vi "Winch v5.vi"() -> ()   [LabVIEW 2013]
uses:
  Globals/Data for Dashboard.vi
  <vilib>/Rock Robotics/WPI/Joystick/WPI_JoystickGetSetRefNum.vi
  Robot Global Data.vi
  Globals/Useful Values.vi
  Globals/Homes.vi
  <vilib>/addons/control/pid/pid.llb/PID (DBL).vi
  <vilib>/Utility/file.llb/Write To Spreadsheet File (DBL).vi
  <vilib>/addons/control/pid/NI_PID_pid.lvlib
panel:
  out "Selector?":bool
  out "Winch Armed?":bool
  out "Winch Power":bool
  out "Full/half?":bool
  out "Full to Half?":bool
  out "Arm?":bool
  in  "PID gains":T1={"proportional gain (Kc)"=2.75, "integral time (Ti, min)"=0.0, "derivative time (Td, min)"=0.0} {"derivative time (Td, min)" format="%.3f"; "integral time (Ti, min)" format="%.3f"; "proportional gain (Kc)" format="%.3f"}
  # "PULLBACK SPEED NEEDS\nTO BE NEGATIVE OR ELSE"
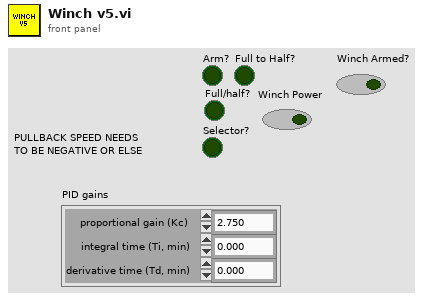
[diagram p1: front panel]
types:
  T1 = cluster{"proportional gain (Kc)":dbl, "integral time (Ti, min)":dbl, "derivative time (Td, min)":dbl}
  T2 = typedef "WPI_DigitalInputDevRef.ctl" = cluster{"DevStatus":errorcluster, "DIO Channel":T3, "Digital Module":T4}
  T3 = typedef "FPGA_DIOChannel.ctl" = enum8{"DIO 1", "DIO 2", "DIO 3", "DIO 4", "DIO 5", "DIO 6", "DIO 7", "DIO 8", "DIO 9", "DIO 10", "DIO 11", "DIO 12", "DIO 13", "DIO 14", "Invalid"}
  T4 = typedef "FPGA_TypedefDigitalModule.ctl" = enum16{"Digital Module 1", "Digital Module 2"}
  T5 = typedef "WPI_MotorControlDeviceRef.ctl" = cluster{"DeviceStatus":errorcluster, "Type":enum16{"PWM", "CAN"}, "PWM":cluster{"Digital Module":T4, "PWM Channel":T6, "DeadBand":T7}, "CAN":cluster{"Device Number":u8, "Control Mode":T8, "Semaphore":T9, "Max Vout":dbl}, "Invert":bool, "TransformRef":T10, "InvTransformRef":T10}
  T6 = typedef "FPGA_DIOPWMChannel.ctl" = enum8{"PWM 1", "PWM 2", "PWM 3", "PWM 4", "PWM 5", "PWM 6", "PWM 7", "PWM 8", "PWM 9", "PWM 10", "Invalid"}
  T7 = typedef "WPI_PWMDeadband.ctl" = cluster{"Name":string, "maxPositivePwm":i32, "minPositivePwm":i32, "centerPwm":i32, "maxNegativePwm":i32, "minNegativePwm":i32, "angularRange":u16}
  T8 = typedef "WPI_CANJaguar_ControlMode.ctl" = enum8{"Percent VBus", "Current", "Speed", "Position", "Voltage"}
  T9 = typedef "Semaphore RefNum" = refnum<k1>
  T10 = typedef "WPI_PWMTransform_ConPane.ctl" = refnum<vi>
  T11 = typedef "WPI_JoystickDevRef.ctl" = cluster{"Device":T12}
  T12 = typedef "WPI_JoystickDeviceEnum.ctl" = enum16{"USB 1", "USB 2", "USB 3", "USB 4", "Kinect 1", "Kinect 2"}
  T13 = typedef "WPI_AnalogChannelDevRef.ctl" = cluster{"DevStatus":errorcluster, "Analog Module":T14, "Analog Channel":T15}
  T14 = typedef "FPGA_TypedefAnalogModule.ctl" = enum16{"Analog Module 1", "Analog Module 2"}
  T15 = typedef "FPGA_AIChannel.ctl" = enum8{"AI 1", "AI 2", "AI 3", "AI 4", "AI 5", "AI 6", "AI 7", "AI 8", "Invalid"}
  T16 = typedef "WPI_DriverStationRobotMode2.ctl" = enum16{"Autonomous Disabled", "Autonomous Enabled", "Teleop Disabled", "Teleop Enabled", "Timeout", "Finish", "Test Disabled", "Test Enabled"}
  T17 = typedef "WPI_JoystickButtonState.ctl" = cluster{"Button 1":bool, "Button 2":bool, "Button 3":bool, "Button 4":bool, "Button 5":bool, "Button 6":bool, "Button 7":bool, "Button 8":bool, "Button 9":bool, "Button 10":bool, "Button 11":bool, "Button 12":bool}
  T18 = cluster{"axis 1 (x)":dbl, "axis 2 (y)":dbl, "axis 3 (throttle)":dbl, "axis 4":dbl, "axis 5":dbl, "axis 6":dbl}
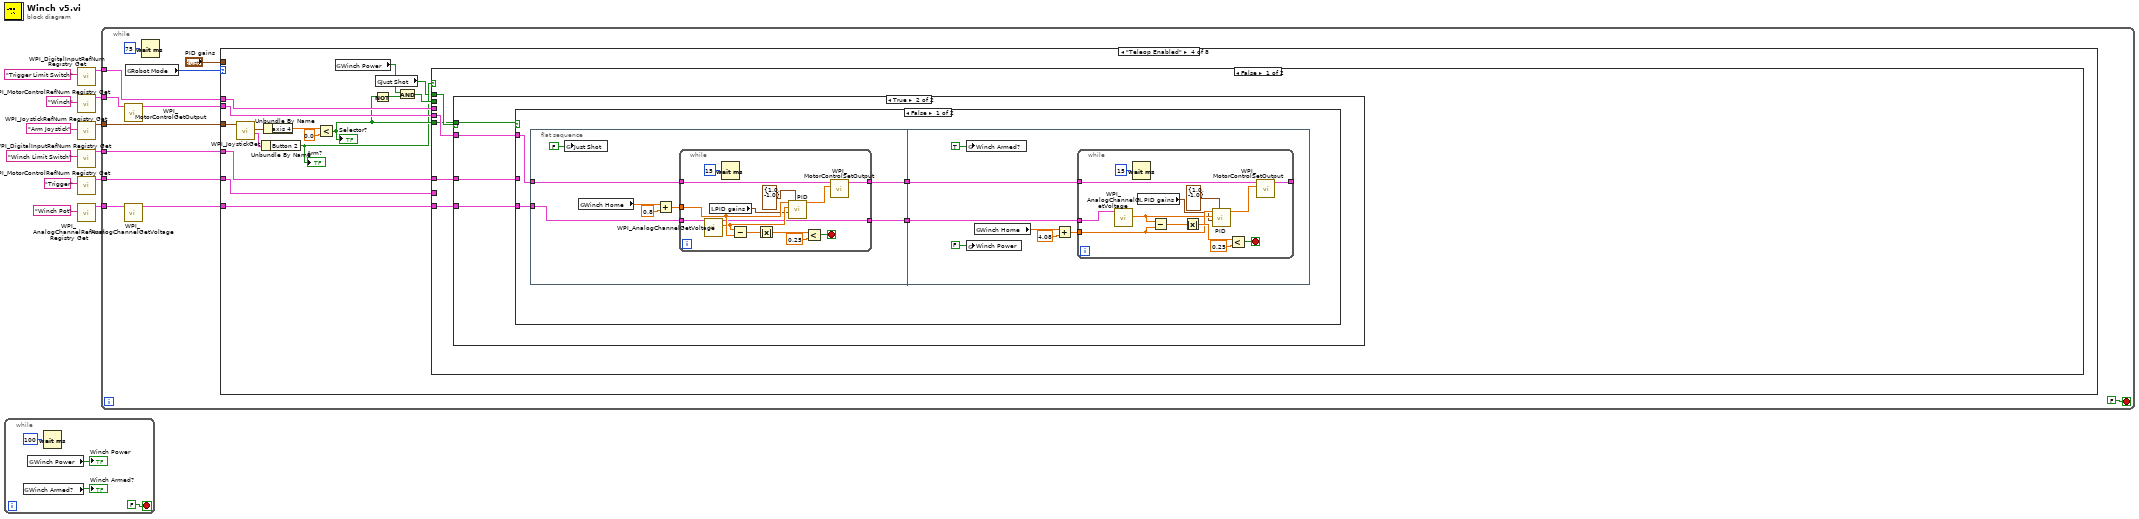
[diagram p0: block diagram]
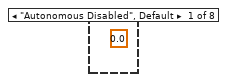
[diagram p2: hidden frame]
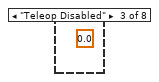
[diagram p4: hidden frame]
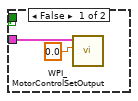
[diagram p5: hidden frame]
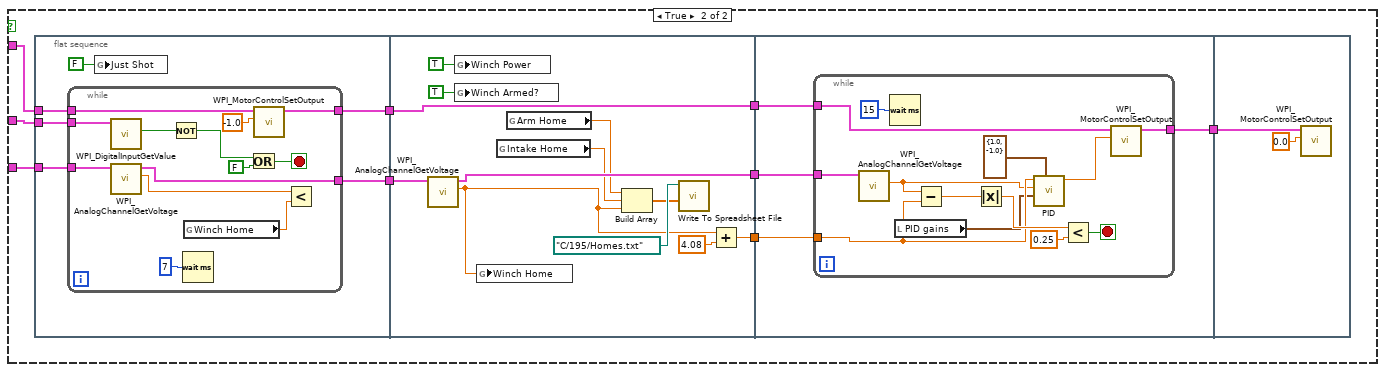
[diagram p6: hidden frame]
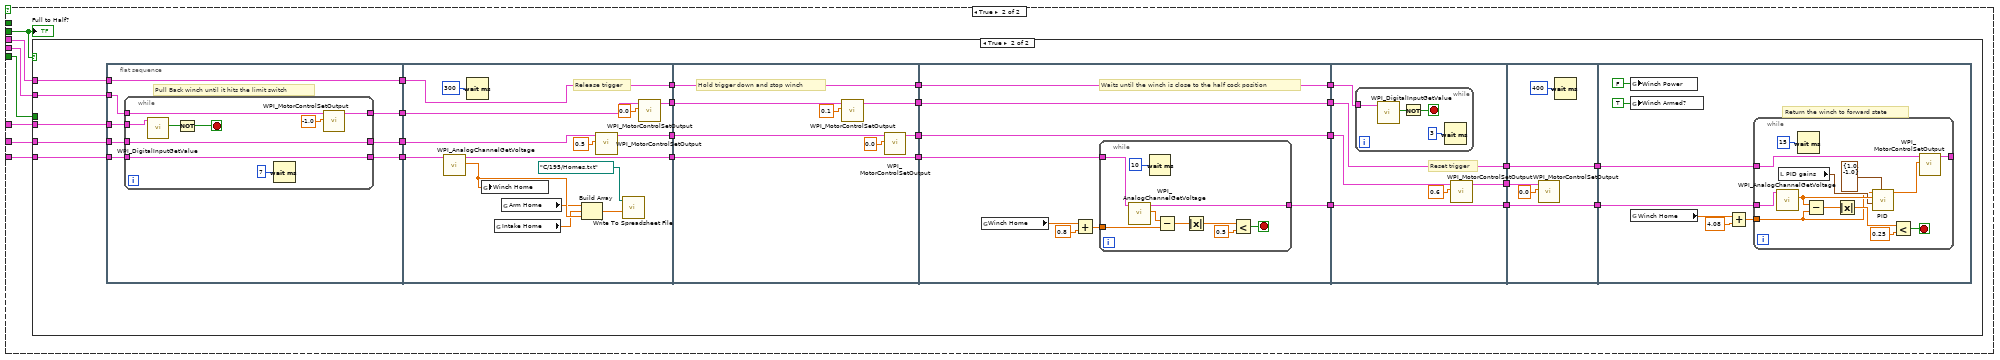
[diagram p7: hidden frame]
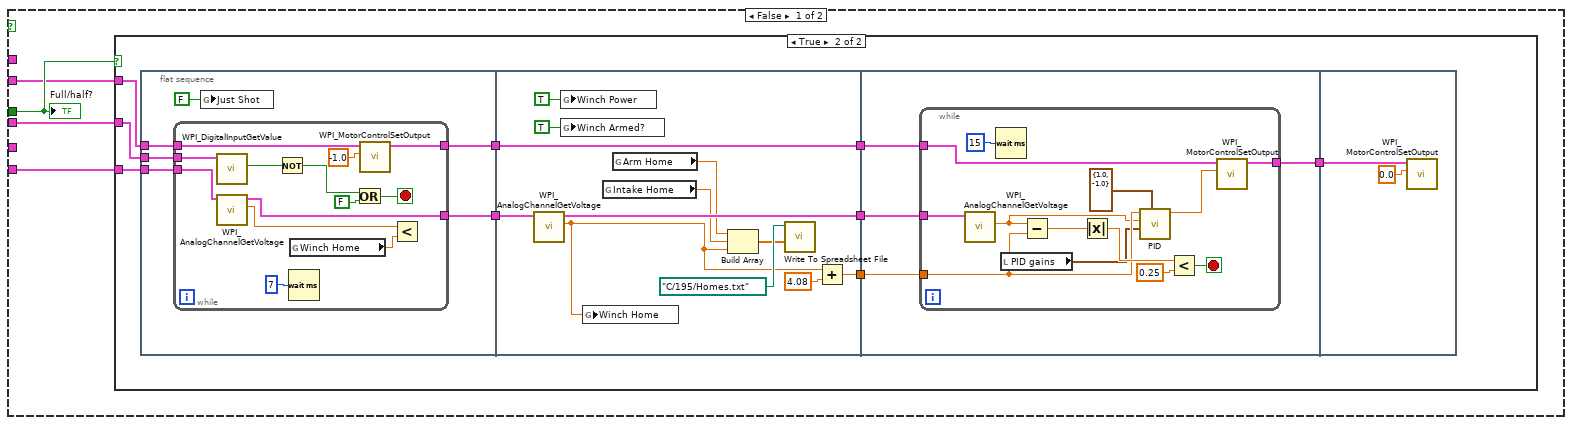
[diagram p8: hidden frame]
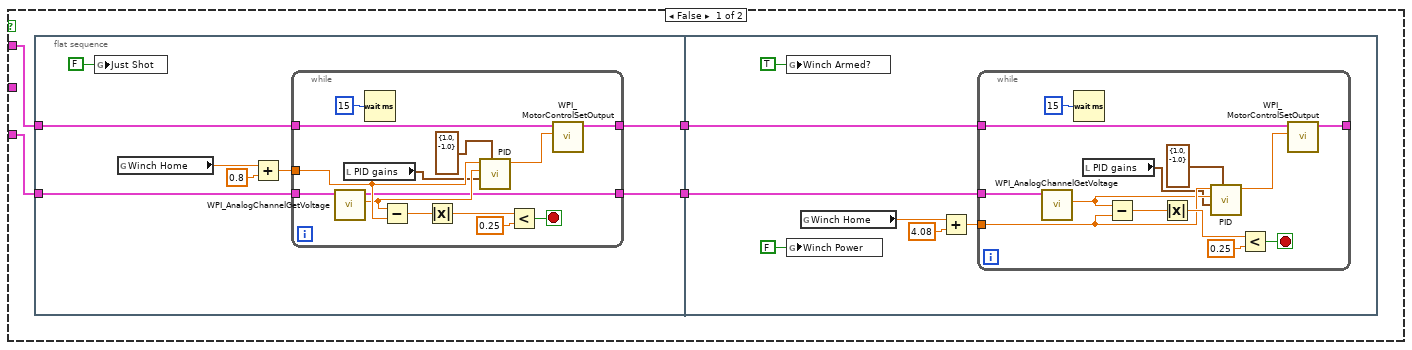
[diagram p9: hidden frame]
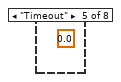
[diagram p10: hidden frame]
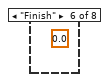
[diagram p11: hidden frame]
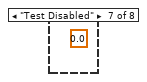
[diagram p12: hidden frame]
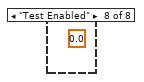
[diagram p13: hidden frame]
diagram:
  n1 = while {
    stop <- FALSE stop-if-true
    n2 = global read "Data for Dashboard.vi" "Winch Armed?"() -> (→"Winch Armed?":bool)
    n3 = global read "Data for Dashboard.vi" "Winch Power"() -> (→"Winch Power":bool)
    n4 = Wait (ms)(milliseconds to wait=u32 100) -> ()  [unwired: 1 out]
  }
  n5 = call <vilib>:"WPI_DigitalInputRefNum Registry Get.vi"("refnum name"="Trigger Limit Switch") -> ("DigitalInputDevRef"=w1:T2)  [unwired: 9 in, 1 out]
  n6 = call <vilib>:"WPI_MotorControlRefNum Registry Get.vi"("refnum name"="Winch") -> ("MotorControlDevRef"=w9:T5)  [unwired: 9 in, 1 out]
  n7 = call <vilib>:"WPI_JoystickRefNum Registry Get.vi"("refnum name"="Arm Joystick") -> ("JoystickDevRef"=w7:T11)  [unwired: 9 in, 1 out]
  n8 = call <vilib>:"WPI_DigitalInputRefNum Registry Get.vi"("refnum name"="Winch Limit Switch") -> ("DigitalInputDevRef"=w6:T2)  [unwired: 9 in, 1 out]
  n9 = call <vilib>:"WPI_MotorControlRefNum Registry Get.vi"("refnum name"="Trigger") -> ("MotorControlDevRef"=w3:T5)  [unwired: 9 in, 1 out]
  n10 = call <vilib>:"WPI_AnalogChannelRefNum Registry Get.vi"("refnum name"="Winch Pot") -> ("AIDeviceRef"=w12:T13)  [unwired: 9 in, 1 out]
  n11 = while {
    tunnel: w12 -> [w26]
    tunnel: w9 -> [w21]
    tunnel: w7 -> [w23]
    tunnel: w6 -> [w18]
    tunnel: w3 -> [w19]
    tunnel: w1 -> [w17]
    stop <- FALSE stop-if-true
    n12 = call <vilib>:"WPI_MotorControlGetOutput.vi"("MotorControlDevRef"=w21) -> ("MotorControlDevRef"=w20:T5)  [unwired: 8 in, 2 out]
    n13 = call <vilib>:"WPI_AnalogChannelGetVoltage.vi"("AIDeviceRef"=w26) -> ("AIDeviceRef"=w22:T13)  [unwired: 8 in, 2 out]
    n14 = global read "Robot Global Data.vi" "Robot Mode"() -> (w25:T16)
    n15 = Wait (ms)(milliseconds to wait=u32 75) -> ()  [unwired: 1 out]
    n16 = case shown="\"Teleop Enabled\"" w25 {
      tunnel: w20 -> [_ _ _ w41 _ _ _ _]
      tunnel: "PID gains" -> [_ _ _ _ _ _ _ _]
      tunnel: w23 -> [_ _ _ w44 _ _ _ _]
      tunnel: w18 -> [_ _ _ w42 _ _ _ _]
      tunnel: w22 -> [_ _ _ w40 _ _ _ _]
      tunnel: w19 -> [_ _ _ w39 _ _ _ _]
      tunnel: w17 -> [_ _ _ w38 _ _ _ _]
      frame "Autonomous Disabled", Default {
        (unwired) 0.0 ("Motor Output")
      }
      frame "Autonomous Enabled" {
      }
      frame "Teleop Disabled" {
        (unwired) 0.0 ("Motor Output")
      }
      frame "Teleop Enabled" {
        n17 = call <vilib>:"WPI_JoystickGet.vi"("JoystickDevRef"=w44) -> ("Buttons"=w43:T17, "Axes"=w35:T18)  [unwired: 4 in, 1 out]
        n18 = Unbundle By Name(w43) -> ("Button 2"=w30:bool)
        "Arm?" <- w30
        n19 = Unbundle By Name(w35) -> ("axis 4"=w34:dbl)
        n20 = Less?(x=w34, y=0.0) -> (x < y?=w32:bool)
        "Selector?" <- w32
        n21 = global read "Data for Dashboard.vi" "Winch Power"() -> (w36:bool)
        n22 = Not(x=w32) -> (.not. x?=w31:bool)
        n23 = global read "Useful Values.vi" "Just Shot"() -> (w29:bool)
        n24 = And(x=w36, y=w31) -> (x .and. y?=w37:bool)
        n25 = case shown="False" w30 {
          tunnel: w42 -> [w47 w165]
          tunnel: w41 -> [w49 w167]
          tunnel: w40 -> [w46 w166]
          tunnel: w39 -> [_ w164]
          tunnel: w38 -> [_ w163]
          tunnel: w37 -> [_ w162]
          tunnel: w32 -> [w45 w161]
          tunnel: w29 -> [w48 _]
          frame False {
            n26 = case shown="True" w48 {
              tunnel: w49 -> [w51 w54]
              tunnel: w47 -> [_ w55]
              tunnel: w46 -> [_ w53]
              tunnel: w45 -> [_ w52]
              frame False {
                n27 = call <vilib>:"WPI_MotorControlSetOutput.vi"("Output"=0.0, "MotorControlDevRef"=w51) -> ()  [unwired: 7 in, 3 out]
              }
              frame True {
                n28 = case shown="False" w52 {
                  tunnel: w54 -> [w58 w104]
                  tunnel: w53 -> [w59 w103]
                  tunnel: w55 -> [_ w102]
                  frame False {
                    n29 = flat-sequence {
                      tunnel: w58 -> [w67]
                      tunnel: w59 -> [w66]
                      tunnel: [w62] -> w57
                      tunnel: [w61] -> w56
                      tunnel: w57 -> [w88]
                      tunnel: w56 -> [w87]
                      frame #0 {
                        n30 = global write "Useful Values.vi" "Just Shot"(FALSE ("Just Shot")) -> ()
                        n31 = global read "Homes.vi" "Winch Home"() -> (w65:dbl)
                        n32 = Add(x=w65, y=0.8) -> (x+y=w63:dbl)
                        n33 = while {
                          tunnel: w67 -> [w81]
                          tunnel: w63 -> [w74]
                          tunnel: w66 -> [w76]
                          tunnel: [w72] -> w62
                          tunnel: [w68] -> w61
                          stop <- w78 stop-if-true
                          n34 = call <vilib>:"WPI_AnalogChannelGetVoltage.vi"("AIDeviceRef"=w76) -> ("Voltage"=w73:dbl, "AIDeviceRef"=w68:T13)  [unwired: 8 in, 1 out]
                          n35 = local read "PID gains"() -> (w71:T1)
                          n36 = Wait (ms)(milliseconds to wait=u32 15) -> ()  [unwired: 1 out]
                          n37 = Subtract(x=w73, y=w74) -> (x-y=w80:dbl)
                          n38 = Absolute Value(x=w80) -> (abs(x)=w79:dbl)
                          n39 = call-poly <vilib>:"PID.vi"("output range"=cluster{"output high":dbl, "output low":dbl} {"output high"=1.0, "output low"=-1.0}, "PID gains"=w71, "process variable"=w73, "setpoint"=w74) -> ("output"=w69:dbl)  [unwired: 6 in, 1 out]
                          n40 = Less?(x=w79, y=0.25) -> (x < y?=w78:bool)
                          n41 = call <vilib>:"WPI_MotorControlSetOutput.vi"("Output"=w69, "MotorControlDevRef"=w81) -> ("MotorControlDevRef"=w72:T5)  [unwired: 7 in, 2 out]
                        }
                      }
                      frame #1 {
                        n42 = global write "Data for Dashboard.vi" "Winch Armed?"(TRUE ("Loaded")) -> ()
                        n43 = global write "Data for Dashboard.vi" "Winch Power"(FALSE ("Loaded")) -> ()
                        n44 = global read "Homes.vi" "Winch Home"() -> (w86:dbl)
                        n45 = Add(x=w86, y=4.08) -> (x+y=w84:dbl)
                        n46 = while {
                          tunnel: w88 -> [w101]
                          tunnel: w84 -> [w94]
                          tunnel: w87 -> [w96]
                          tunnel: [w92] -> _
                          stop <- w98 stop-if-true
                          n47 = call <vilib>:"WPI_AnalogChannelGetVoltage.vi"("AIDeviceRef"=w96) -> ("Voltage"=w93:dbl)  [unwired: 8 in, 2 out]
                          n48 = Wait (ms)(milliseconds to wait=u32 15) -> ()  [unwired: 1 out]
                          n49 = local read "PID gains"() -> (w91:T1)
                          n50 = Subtract(x=w93, y=w94) -> (x-y=w100:dbl)
                          n51 = Absolute Value(x=w100) -> (abs(x)=w99:dbl)
                          n52 = call-poly <vilib>:"PID.vi"("output range"=cluster{"output high":dbl, "output low":dbl} {"output high"=1.0, "output low"=-1.0}, "PID gains"=w91, "process variable"=w93, "setpoint"=w94) -> ("output"=w89:dbl)  [unwired: 6 in, 1 out]
                          n53 = Less?(x=w99, y=0.25) -> (x < y?=w98:bool)
                          n54 = call <vilib>:"WPI_MotorControlSetOutput.vi"("Output"=w89, "MotorControlDevRef"=w101) -> ("MotorControlDevRef"=w92:T5)  [unwired: 7 in, 2 out]
                        }
                      }
                    }
                  }
                  frame True {
                    n55 = flat-sequence {
                      tunnel: w102 -> [w116]
                      tunnel: w104 -> [w115]
                      tunnel: [w114] -> w110
                      tunnel: [w111] -> w109
                      tunnel: w103 -> [w112]
                      tunnel: w110 -> [w141]
                      tunnel: [w141] -> w108
                      tunnel: [w140] -> w107
                      tunnel: w109 -> [w139]
                      tunnel: [w138] -> w106
                      tunnel: w108 -> [w145]
                      tunnel: w107 -> [w143]
                      tunnel: [w142] -> w105
                      tunnel: w106 -> [w144]
                      tunnel: w105 -> [w160]
                      frame #0 {
                        n56 = while {
                          tunnel: w116 -> [w129]
                          tunnel: w115 -> [w125]
                          tunnel: [w124] -> w114
                          tunnel: w112 -> [w123]
                          tunnel: [w122] -> w111
                          stop <- w119 stop-if-true
                          n57 = call <vilib>:"WPI_DigitalInputGetValue.vi"("DigitalInputDevRef"=w129) -> ("Value"=w128:bool)  [unwired: 8 in, 2 out]
                          n58 = call <vilib>:"WPI_AnalogChannelGetVoltage.vi"("AIDeviceRef"=w123) -> ("Voltage"=w121:dbl, "AIDeviceRef"=w122:T13)  [unwired: 8 in, 1 out]
                          n59 = Not(x=w128) -> (.not. x?=w118:bool)
                          n60 = Wait (ms)(milliseconds to wait=u32 7) -> ()  [unwired: 1 out]
                          n61 = global read "Homes.vi" "Winch Home"() -> (w120:dbl)
                          n62 = Or(x=w118, y=FALSE) -> (x .or. y?=w119:bool)
                          n63 = call <vilib>:"WPI_MotorControlSetOutput.vi"("Output"=-1.0 ("Pullback Speed"), "MotorControlDevRef"=w125) -> ("MotorControlDevRef"=w124:T5)  [unwired: 7 in, 2 out]
                          n64 = Less?(x=w121, y=w120) -> ()  [unwired: 1 out]
                        }
                        n65 = global write "Useful Values.vi" "Just Shot"(FALSE ("Just Shot")) -> ()
                      }
                      frame #1 {
                        n66 = call <vilib>:"WPI_AnalogChannelGetVoltage.vi"("AIDeviceRef"=w139) -> ("Voltage"=w132:dbl, "AIDeviceRef"=w140:T13)  [unwired: 8 in, 1 out]
                        n67 = global write "Data for Dashboard.vi" "Winch Power"(TRUE ("Loaded")) -> ()
                        n68 = global write "Data for Dashboard.vi" "Winch Armed?"(TRUE ("Loaded")) -> ()
                        n69 = global write "Homes.vi" "Winch Home"(w132) -> ()
                        n70 = global read "Homes.vi" "Intake Home"() -> (w133:dbl)
                        n71 = global read "Homes.vi" "Arm Home"() -> (w135:dbl)
                        n72 = Build Array(w135, w133, w132) -> (w134:dbl[])
                        n73 = call-poly <vilib>:"Write To Spreadsheet File.vi"("1D data"=w134, "file path (dialog if empty)"=path "C:/195/Homes.txt") -> ()  [unwired: 6 in, 1 out]
                        n74 = Add(x=w132, y=4.08) -> (x+y=w138:dbl)
                      }
                      frame #2 {
                        n75 = while {
                          tunnel: w145 -> [w158]
                          tunnel: w144 -> [w151]
                          tunnel: w143 -> [w153]
                          tunnel: [w149] -> w142
                          stop <- w155 stop-if-true
                          n76 = call <vilib>:"WPI_AnalogChannelGetVoltage.vi"("AIDeviceRef"=w153) -> ("Voltage"=w150:dbl)  [unwired: 8 in, 2 out]
                          n77 = Wait (ms)(milliseconds to wait=u32 15) -> ()  [unwired: 1 out]
                          n78 = local read "PID gains"() -> (w148:T1)
                          n79 = Subtract(x=w150, y=w151) -> (x-y=w157:dbl)
                          n80 = Absolute Value(x=w157) -> (abs(x)=w156:dbl)
                          n81 = call-poly <vilib>:"PID.vi"("output range"=cluster{"output high":dbl, "output low":dbl} {"output high"=1.0, "output low"=-1.0}, "PID gains"=w148, "process variable"=w150, "setpoint"=w151) -> ("output"=w146:dbl)  [unwired: 6 in, 1 out]
                          n82 = Less?(x=w156, y=0.25) -> (x < y?=w155:bool)
                          n83 = call <vilib>:"WPI_MotorControlSetOutput.vi"("Output"=w146, "MotorControlDevRef"=w158) -> ("MotorControlDevRef"=w149:T5)  [unwired: 7 in, 2 out]
                        }
                      }
                      frame #3 {
                        n84 = call <vilib>:"WPI_MotorControlSetOutput.vi"("Output"=0.0, "MotorControlDevRef"=w160) -> ()  [unwired: 7 in, 3 out]
                      }
                    }
                  }
                }
              }
            }
          }
          frame True {
            n85 = case shown="True" w162 {
              tunnel: w167 -> [w170 w281]
              tunnel: w166 -> [w169 w280]
              tunnel: w165 -> [w168 w279]
              tunnel: w164 -> [_ w278]
              tunnel: w163 -> [_ w277]
              tunnel: w161 -> [w171 _]
              frame False {
                n86 = case shown="True" w171 {
                  tunnel: w170 -> [w174 w220]
                  tunnel: w169 -> [w175 w219]
                  tunnel: w168 -> [_ w218]
                  frame False {
                    n87 = flat-sequence {
                      tunnel: w174 -> [w183]
                      tunnel: w175 -> [w182]
                      tunnel: [w178] -> w173
                      tunnel: [w177] -> w172
                      tunnel: w173 -> [w204]
                      tunnel: w172 -> [w203]
                      frame #0 {
                        n88 = global write "Useful Values.vi" "Just Shot"(FALSE ("Just Shot")) -> ()
                        n89 = global read "Homes.vi" "Winch Home"() -> (w181:dbl)
                        n90 = Add(x=w181, y=0.8) -> (x+y=w179:dbl)
                        n91 = while {
                          tunnel: w183 -> [w197]
                          tunnel: w179 -> [w190]
                          tunnel: w182 -> [w192]
                          tunnel: [w188] -> w178
                          tunnel: [w184] -> w177
                          stop <- w194 stop-if-true
                          n92 = call <vilib>:"WPI_AnalogChannelGetVoltage.vi"("AIDeviceRef"=w192) -> ("Voltage"=w189:dbl, "AIDeviceRef"=w184:T13)  [unwired: 8 in, 1 out]
                          n93 = local read "PID gains"() -> (w187:T1)
                          n94 = Wait (ms)(milliseconds to wait=u32 15) -> ()  [unwired: 1 out]
                          n95 = Subtract(x=w189, y=w190) -> (x-y=w196:dbl)
                          n96 = Absolute Value(x=w196) -> (abs(x)=w195:dbl)
                          n97 = call-poly <vilib>:"PID.vi"("output range"=cluster{"output high":dbl, "output low":dbl} {"output high"=1.0, "output low"=-1.0}, "PID gains"=w187, "process variable"=w189, "setpoint"=w190) -> ("output"=w185:dbl)  [unwired: 6 in, 1 out]
                          n98 = Less?(x=w195, y=0.25) -> (x < y?=w194:bool)
                          n99 = call <vilib>:"WPI_MotorControlSetOutput.vi"("Output"=w185, "MotorControlDevRef"=w197) -> ("MotorControlDevRef"=w188:T5)  [unwired: 7 in, 2 out]
                        }
                      }
                      frame #1 {
                        n100 = global write "Data for Dashboard.vi" "Winch Armed?"(TRUE ("Loaded")) -> ()
                        n101 = global write "Data for Dashboard.vi" "Winch Power"(FALSE ("Loaded")) -> ()
                        n102 = global read "Homes.vi" "Winch Home"() -> (w202:dbl)
                        n103 = Add(x=w202, y=4.08) -> (x+y=w200:dbl)
                        n104 = while {
                          tunnel: w204 -> [w217]
                          tunnel: w200 -> [w210]
                          tunnel: w203 -> [w212]
                          tunnel: [w208] -> _
                          stop <- w214 stop-if-true
                          n105 = call <vilib>:"WPI_AnalogChannelGetVoltage.vi"("AIDeviceRef"=w212) -> ("Voltage"=w209:dbl)  [unwired: 8 in, 2 out]
                          n106 = Wait (ms)(milliseconds to wait=u32 15) -> ()  [unwired: 1 out]
                          n107 = local read "PID gains"() -> (w207:T1)
                          n108 = Subtract(x=w209, y=w210) -> (x-y=w216:dbl)
                          n109 = Absolute Value(x=w216) -> (abs(x)=w215:dbl)
                          n110 = call-poly <vilib>:"PID.vi"("output range"=cluster{"output high":dbl, "output low":dbl} {"output high"=1.0, "output low"=-1.0}, "PID gains"=w207, "process variable"=w209, "setpoint"=w210) -> ("output"=w205:dbl)  [unwired: 6 in, 1 out]
                          n111 = Less?(x=w215, y=0.25) -> (x < y?=w214:bool)
                          n112 = call <vilib>:"WPI_MotorControlSetOutput.vi"("Output"=w205, "MotorControlDevRef"=w217) -> ("MotorControlDevRef"=w208:T5)  [unwired: 7 in, 2 out]
                        }
                      }
                    }
                  }
                  frame True {
                    n113 = flat-sequence {
                      tunnel: w218 -> [w232]
                      tunnel: w220 -> [w231]
                      tunnel: [w230] -> w226
                      tunnel: [w227] -> w225
                      tunnel: w219 -> [w228]
                      tunnel: w226 -> [w257]
                      tunnel: [w257] -> w224
                      tunnel: [w256] -> w223
                      tunnel: w225 -> [w255]
                      tunnel: [w254] -> w222
                      tunnel: w224 -> [w261]
                      tunnel: w223 -> [w259]
                      tunnel: [w258] -> w221
                      tunnel: w222 -> [w260]
                      tunnel: w221 -> [w276]
                      frame #0 {
                        n114 = while {
                          tunnel: w232 -> [w245]
                          tunnel: w231 -> [w241]
                          tunnel: [w240] -> w230
                          tunnel: w228 -> [w239]
                          tunnel: [w238] -> w227
                          stop <- w235 stop-if-true
                          n115 = call <vilib>:"WPI_DigitalInputGetValue.vi"("DigitalInputDevRef"=w245) -> ("Value"=w244:bool)  [unwired: 8 in, 2 out]
                          n116 = call <vilib>:"WPI_AnalogChannelGetVoltage.vi"("AIDeviceRef"=w239) -> ("Voltage"=w237:dbl, "AIDeviceRef"=w238:T13)  [unwired: 8 in, 1 out]
                          n117 = Not(x=w244) -> (.not. x?=w234:bool)
                          n118 = Wait (ms)(milliseconds to wait=u32 7) -> ()  [unwired: 1 out]
                          n119 = global read "Homes.vi" "Winch Home"() -> (w236:dbl)
                          n120 = Or(x=w234, y=FALSE) -> (x .or. y?=w235:bool)
                          n121 = call <vilib>:"WPI_MotorControlSetOutput.vi"("Output"=-1.0 ("Pullback Speed"), "MotorControlDevRef"=w241) -> ("MotorControlDevRef"=w240:T5)  [unwired: 7 in, 2 out]
                          n122 = Less?(x=w237, y=w236) -> ()  [unwired: 1 out]
                        }
                        n123 = global write "Useful Values.vi" "Just Shot"(FALSE ("Just Shot")) -> ()
                      }
                      frame #1 {
                        n124 = call <vilib>:"WPI_AnalogChannelGetVoltage.vi"("AIDeviceRef"=w255) -> ("Voltage"=w248:dbl, "AIDeviceRef"=w256:T13)  [unwired: 8 in, 1 out]
                        n125 = global write "Data for Dashboard.vi" "Winch Power"(TRUE ("Loaded")) -> ()
                        n126 = global write "Data for Dashboard.vi" "Winch Armed?"(TRUE ("Loaded")) -> ()
                        n127 = global write "Homes.vi" "Winch Home"(w248) -> ()
                        n128 = global read "Homes.vi" "Intake Home"() -> (w249:dbl)
                        n129 = global read "Homes.vi" "Arm Home"() -> (w251:dbl)
                        n130 = Build Array(w251, w249, w248) -> (w250:dbl[])
                        n131 = call-poly <vilib>:"Write To Spreadsheet File.vi"("1D data"=w250, "file path (dialog if empty)"=path "C:/195/Homes.txt") -> ()  [unwired: 6 in, 1 out]
                        n132 = Add(x=w248, y=4.08) -> (x+y=w254:dbl)
                      }
                      frame #2 {
                        n133 = while {
                          tunnel: w261 -> [w274]
                          tunnel: w260 -> [w267]
                          tunnel: w259 -> [w269]
                          tunnel: [w265] -> w258
                          stop <- w271 stop-if-true
                          n134 = call <vilib>:"WPI_AnalogChannelGetVoltage.vi"("AIDeviceRef"=w269) -> ("Voltage"=w266:dbl)  [unwired: 8 in, 2 out]
                          n135 = Wait (ms)(milliseconds to wait=u32 15) -> ()  [unwired: 1 out]
                          n136 = local read "PID gains"() -> (w264:T1)
                          n137 = Subtract(x=w266, y=w267) -> (x-y=w273:dbl)
                          n138 = Absolute Value(x=w273) -> (abs(x)=w272:dbl)
                          n139 = call-poly <vilib>:"PID.vi"("output range"=cluster{"output high":dbl, "output low":dbl} {"output high"=1.0, "output low"=-1.0}, "PID gains"=w264, "process variable"=w266, "setpoint"=w267) -> ("output"=w262:dbl)  [unwired: 6 in, 1 out]
                          n140 = Less?(x=w272, y=0.25) -> (x < y?=w271:bool)
                          n141 = call <vilib>:"WPI_MotorControlSetOutput.vi"("Output"=w262, "MotorControlDevRef"=w274) -> ("MotorControlDevRef"=w265:T5)  [unwired: 7 in, 2 out]
                        }
                      }
                      frame #3 {
                        n142 = call <vilib>:"WPI_MotorControlSetOutput.vi"("Output"=0.0, "MotorControlDevRef"=w276) -> ()  [unwired: 7 in, 3 out]
                      }
                    }
                  }
                }
                "Full/half?" <- w171
              }
              frame True {
                n143 = flat-sequence {
                  tunnel: w281 -> [w310]
                  tunnel: w280 -> [w309]
                  tunnel: w279 -> [w308]
                  tunnel: w278 -> [w306]
                  tunnel: [w307] -> w302
                  tunnel: [w305] -> w301
                  tunnel: [w304] -> w300
                  tunnel: [w303] -> w299
                  tunnel: w277 -> [w303]
                  tunnel: w302 -> [w334]
                  tunnel: [w331] -> w298
                  tunnel: [w320] -> w297
                  tunnel: w301 -> [w322]
                  tunnel: w300 -> [w324]
                  tunnel: [w323] -> w296
                  tunnel: [w330] -> w295
                  tunnel: w299 -> [w330]
                  tunnel: w298 -> [w342]
                  tunnel: w297 -> [w339]
                  tunnel: w296 -> [w340]
                  tunnel: [w340] -> w294
                  tunnel: [w338] -> w293
                  tunnel: [w336] -> w292
                  tunnel: w295 -> [w336]
                  tunnel: [w335] -> w291
                  tunnel: w294 -> [w349]
                  tunnel: w293 -> [w350]
                  tunnel: [w350] -> w290
                  tunnel: [w345] -> w289
                  tunnel: w292 -> [w345]
                  tunnel: w291 -> [w344]
                  tunnel: [w344] -> w288
                  tunnel: [w343] -> w287
                  tunnel: w290 -> [w365]
                  tunnel: [w365] -> w286
                  tunnel: w289 -> [w364]
                  tunnel: w288 -> [w362]
                  tunnel: [w361] -> w285
                  tunnel: w287 -> [w360]
                  tunnel: [w360] -> w284
                  tunnel: w286 -> [w374]
                  tunnel: [w374] -> w283
                  tunnel: w285 -> [w370]
                  tunnel: w284 -> [w373]
                  tunnel: [w373] -> w282
                  tunnel: w283 -> [w381]
                  tunnel: w282 -> [w380]
                  frame #0 {
                    # "Pull Back winch until it hits the limit switch"
                    n144 = while {
                      tunnel: [w316] -> w305
                      tunnel: w310 -> [w314]
                      tunnel: w309 -> [w311]
                      tunnel: w308 -> [w313]
                      tunnel: [w312] -> w307
                      tunnel: w306 -> [w312]
                      tunnel: [w311] -> w304
                      stop <- w315 stop-if-true
                      n145 = call <vilib>:"WPI_DigitalInputGetValue.vi"("DigitalInputDevRef"=w313) -> ("Value"=w319:bool)  [unwired: 8 in, 2 out]
                      n146 = Not(x=w319) -> (.not. x?=w315:bool)
                      n147 = Wait (ms)(milliseconds to wait=u32 7) -> ()  [unwired: 1 out]
                      n148 = call <vilib>:"WPI_MotorControlSetOutput.vi"("Output"=-1.0 ("Pullback Speed"), "MotorControlDevRef"=w314) -> ("MotorControlDevRef"=w316:T5)  [unwired: 7 in, 2 out]
                    }
                  }
                  frame #1 {
                    # "Release trigger"
                    n149 = call <vilib>:"WPI_AnalogChannelGetVoltage.vi"("AIDeviceRef"=w324) -> ("Voltage"=w329:dbl, "AIDeviceRef"=w323:T13)  [unwired: 8 in, 1 out]
                    n150 = Wait (ms)(milliseconds to wait=u32 300) -> ()  [unwired: 1 out]
                    n151 = global write "Homes.vi" "Winch Home"(w329) -> ()
                    n152 = global read "Homes.vi" "Intake Home"() -> (w328:dbl)
                    n153 = global read "Homes.vi" "Arm Home"() -> (w326:dbl)
                    n154 = Build Array(w326, w328, w329) -> (w327:dbl[])
                    n155 = call <vilib>:"WPI_MotorControlSetOutput.vi"("Output"=0.5, "MotorControlDevRef"=w334) -> ("MotorControlDevRef"=w331:T5)  [unwired: 7 in, 2 out]
                    n156 = call-poly <vilib>:"Write To Spreadsheet File.vi"("1D data"=w327, "file path (dialog if empty)"=path "C:/195/Homes.txt") -> ()  [unwired: 6 in, 1 out]
                    n157 = call <vilib>:"WPI_MotorControlSetOutput.vi"("Output"=0.0, "MotorControlDevRef"=w322) -> ("MotorControlDevRef"=w320:T5)  [unwired: 7 in, 2 out]
                  }
                  frame #2 {
                    # "Hold trigger down and stop winch"
                    n158 = call <vilib>:"WPI_MotorControlSetOutput.vi"("Output"=0.1, "MotorControlDevRef"=w339) -> ("MotorControlDevRef"=w338:T5)  [unwired: 7 in, 2 out]
                    n159 = call <vilib>:"WPI_MotorControlSetOutput.vi"("Output"=0.0, "MotorControlDevRef"=w342) -> ("MotorControlDevRef"=w335:T5)  [unwired: 7 in, 2 out]
                  }
                  frame #3 {
                    # "Waits until the winch is close to the half cock position"
                    n160 = global read "Homes.vi" "Winch Home"() -> (w348:dbl)
                    n161 = Add(x=w348, y=0.8) -> (x+y=w346:dbl)
                    n162 = while {
                      tunnel: w349 -> [w359]
                      tunnel: w346 -> [w352]
                      tunnel: [w351] -> w343
                      stop <- w353 stop-if-true
                      n163 = call <vilib>:"WPI_AnalogChannelGetVoltage.vi"("AIDeviceRef"=w359) -> ("Voltage"=w358:dbl, "AIDeviceRef"=w351:T13)  [unwired: 8 in, 1 out]
                      n164 = Wait (ms)(milliseconds to wait=u32 10) -> ()  [unwired: 1 out]
                      n165 = Subtract(x=w358, y=w352) -> (x-y=w357:dbl)
                      n166 = Absolute Value(x=w357) -> (abs(x)=w356:dbl)
                      n167 = Less?(x=w356, y=0.5) -> (x < y?=w353:bool)
                    }
                  }
                  frame #4 {
                    # "Reset trigger"
                    n168 = while {
                      tunnel: w364 -> [w369]
                      stop <- w367 stop-if-true
                      n169 = call <vilib>:"WPI_DigitalInputGetValue.vi"("DigitalInputDevRef"=w369) -> ("Value"=w368:bool)  [unwired: 8 in, 2 out]
                      n170 = Not(x=w368) -> (.not. x?=w367:bool)
                      n171 = Wait (ms)(milliseconds to wait=u32 3) -> ()  [unwired: 1 out]
                    }
                    n172 = call <vilib>:"WPI_MotorControlSetOutput.vi"("Output"=0.6, "MotorControlDevRef"=w362) -> ("MotorControlDevRef"=w361:T5)  [unwired: 7 in, 2 out]
                  }
                  frame #5 {
                    n173 = call <vilib>:"WPI_MotorControlSetOutput.vi"("Output"=0.0, "MotorControlDevRef"=w370) -> ()  [unwired: 7 in, 3 out]
                    n174 = Wait (ms)(milliseconds to wait=u32 400) -> ()  [unwired: 1 out]
                  }
                  frame #6 {
                    # "Return the winch to forward state"
                    n175 = global write "Data for Dashboard.vi" "Winch Power"(FALSE ("Loaded")) -> ()
                    n176 = global write "Data for Dashboard.vi" "Winch Armed?"(TRUE ("Loaded")) -> ()
                    n177 = global read "Homes.vi" "Winch Home"() -> (w379:dbl)
                    n178 = Add(x=w379, y=4.08) -> (x+y=w377:dbl)
                    n179 = while {
                      tunnel: w381 -> [w394]
                      tunnel: [w387] -> _
                      tunnel: w380 -> [w383]
                      tunnel: w377 -> [w382]
                      stop <- w391 stop-if-true
                      n180 = call <vilib>:"WPI_AnalogChannelGetVoltage.vi"("AIDeviceRef"=w383) -> ("Voltage"=w388:dbl)  [unwired: 8 in, 2 out]
                      n181 = local read "PID gains"() -> (w386:T1)
                      n182 = Wait (ms)(milliseconds to wait=u32 15) -> ()  [unwired: 1 out]
                      n183 = Subtract(x=w388, y=w382) -> (x-y=w393:dbl)
                      n184 = Absolute Value(x=w393) -> (abs(x)=w392:dbl)
                      n185 = call-poly <vilib>:"PID.vi"("output range"=cluster{"output high":dbl, "output low":dbl} {"output high"=1.0, "output low"=-1.0}, "PID gains"=w386, "process variable"=w388, "setpoint"=w382) -> ("output"=w384:dbl)  [unwired: 6 in, 1 out]
                      n186 = Less?(x=w392, y=0.25) -> (x < y?=w391:bool)
                      n187 = call <vilib>:"WPI_MotorControlSetOutput.vi"("Output"=w384, "MotorControlDevRef"=w394) -> ("MotorControlDevRef"=w387:T5)  [unwired: 7 in, 2 out]
                    }
                  }
                }
              }
            }
            "Full to Half?" <- w162
          }
        }
      }
      frame "Timeout" {
        (unwired) 0.0 ("Motor Output")
      }
      frame "Finish" {
        (unwired) 0.0 ("Motor Output")
      }
      frame "Test Disabled" {
        (unwired) 0.0 ("Motor Output")
      }
      frame "Test Enabled" {
        (unwired) 0.0 ("Motor Output")
      }
    }
  }
